vi "Stop Nested Actors.vi"(8 "Error In":errorcluster, 11 "LHW-GUI-Actor in":refnum<class "LHW-GUI-Actor.lvclass">) -> (0 "Error Out":errorcluster, 3 "LHW-GUI-Actor out":refnum<class "LHW-GUI-Actor.lvclass">)   [LabVIEW 2014, in "LHW-GUI.lvlib" / "LHW-GUI-Actor.lvclass"]
doc: "Stop nested actors."
uses:
  LHW-GUI-Actor.lvclass
  <vilib>/ActorFramework/Message Enqueuer/Message Enqueuer.lvclass
  LHW-GUI-Actor.lvclass/LHW-GUI-Actor.ctl
  <vilib>/ActorFramework/Message Enqueuer/Message Enqueuer.lvclass/Message Enqueuer.ctl
  <vilib>/ActorFramework/Message Enqueuer/Enqueue.vi
  <vilib>/ActorFramework/Message Priority Queue/Priority Enqueue.vi
  <vilib>/ActorFramework/Stop Msg/Stop Msg.lvclass
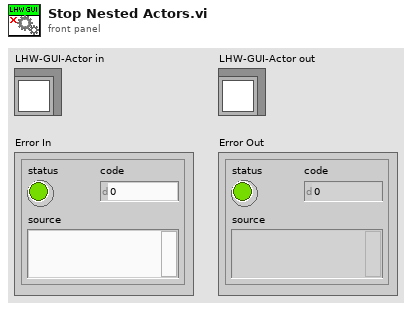
[diagram p1: front panel]
types:
  T1 = cluster{"LHW-Acquisition":refnum<class "Message Enqueuer.lvclass">, "LHW-Analysis":refnum<class "Message Enqueuer.lvclass">, "LHW-Storage":refnum<class "Message Enqueuer.lvclass">}
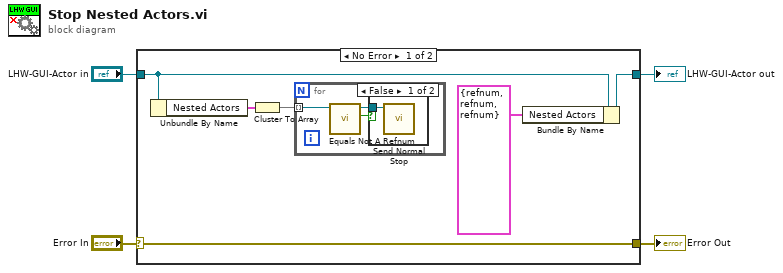
[diagram p0: block diagram]
diagram:
  n1 = case shown="No Error" "Error In" {
    selector: "Error In" -> [w10 w15]
    tunnel: [w10 w15] -> w3
    tunnel: [w5 w14] -> w1
    tunnel: "LHW-GUI-Actor in" -> [w6 w14]
    frame No Error {
      n2 = Unbundle By Name(w6) -> ("Nested Actors"=w9:T1)
      n3 = Cluster To Array(cluster=w9) -> (array=w8:refnum<class "Message Enqueuer.lvclass">[])
      n4 = for {
        tunnel: w8 -> [w12] mode=indexing
        n5 = call <vilib>:"Equals Not A Refnum.vi"("Message Enqueuer"=w12) -> ("Not a refnum?"=w11:bool)  [unwired: 10 in]
        n6 = case shown="False" w11 {
          tunnel: w12 -> [w13 _]
          frame False {
            n7 = call <vilib>:"Send Normal Stop.vi"("Message Enqueuer"=w13) -> ()  [unwired: 10 in, 1 out]
          }
          frame True {
          }
        }
      }
      n8 = Bundle By Name(cluster=w6, "Nested Actors"=T1 {"LHW-Acquisition"=refnum, "LHW-Analysis"=refnum, "LHW-Storage"=refnum}) -> (w5:refnum<class "LHW-GUI-Actor.lvclass">)
    }
    frame Error {
    }
  }
  "Error Out" <- w3
  "LHW-GUI-Actor out" <- w1
